vi "Resistance of the Helium Probe (Set).vi"(6 "ISOBUS address":T4=-1 caption="ISOBUS address (-1)", 8 "error in":errorcluster, 9 "Unit":T1, 10 "Resistance Configuration":T5, 11 "Mercury Reference In":T6) -> (0 "error out":errorcluster, 2 "Response":T2, 3 "Mercury Reference Out":T6, 4 "Valid?":T3)   [LabVIEW 2015, in "Mercury iXX.lvlib" / "Level Meter.lvlib"]
doc: "Set the configuration for the resistance of the helium probe at both 0% and 100%."
uses:
  Level Meter.lvlib
  Controls/Mercury Reference.ctl
  Controls/Comms Transport Layer.ctl
  Private/Controls/Query Dynamic Reference.ctl
  Controls/Resistance Configuration.ctl
  Controls/ISOBus Address.ctl
  Controls/Is Valid LED.ctl
  Controls/Response String.ctl
  Controls/Unit String.ctl
  Private/Controls/Command Verbs.ctl
  Mercury iXX.lvlib
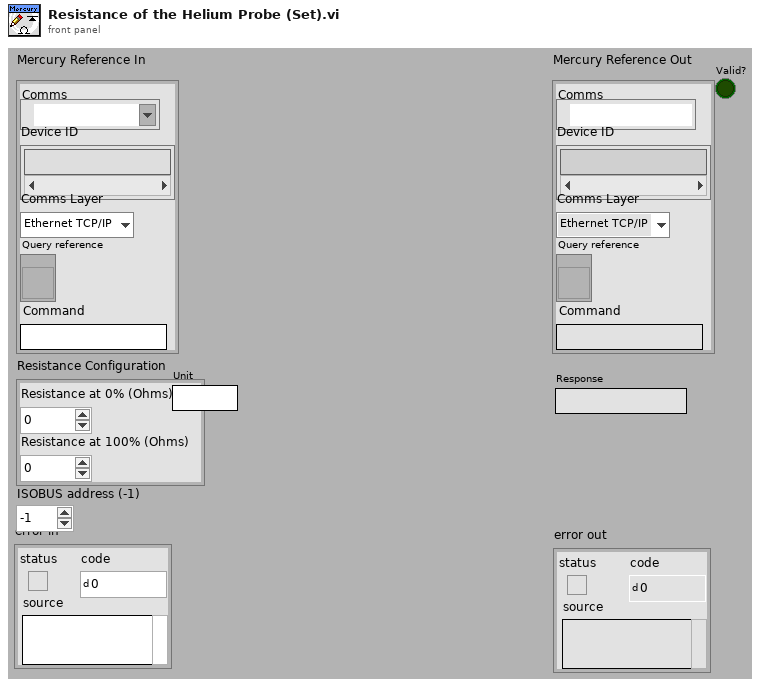
[diagram p1: front panel]
types:
  T1 = typedef "Mercury iXX.lvlib/Unit String.ctl" = string
  T2 = typedef "Mercury iXX.lvlib/Response String.ctl" = string
  T3 = typedef "Mercury iXX.lvlib/Is Valid LED.ctl" = bool
  T4 = typedef "Mercury iXX.lvlib/ISOBus Address.ctl" = i32
  T5 = typedef "Mercury iXX.lvlib/Level Meter.lvlib/Resistance Configuration.ctl" = cluster{"Res 0%":dbl, "Res 100%":dbl}
  T6 = typedef "Mercury iXX.lvlib/Mercury Reference.ctl" = cluster{"Comms":refnum<visa-resource-name>, "Device ID":string[], "Comms Layer":T7, "Command":string, "Query reference":T8}
  T7 = typedef "Mercury iXX.lvlib/Comms Transport Layer.ctl" = enum16{"Ethernet TCP/IP", "USB", "ISOBus - RS-232", "GPIB"}
  T8 = typedef "Mercury iXX.lvlib/Query Dynamic Reference.ctl" = refnum<vi>
  T9 = typedef "Mercury iXX.lvlib/Command Verbs.ctl" = string
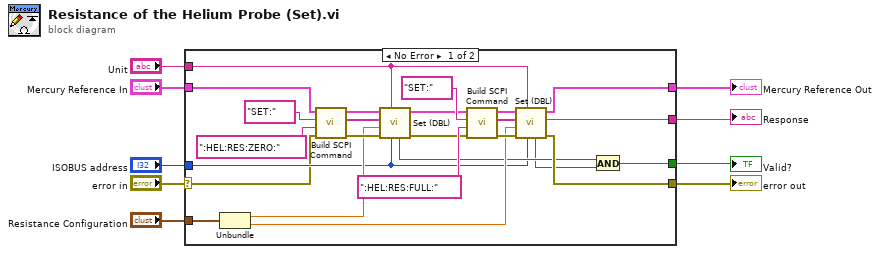
[diagram p0: block diagram]
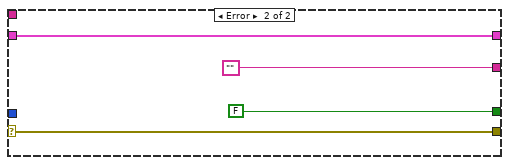
[diagram p2: hidden frame]
diagram:
  n1 = case shown="No Error" "error in" {
    selector: "error in" -> [w11 w38]
    tunnel: "Resistance Configuration" -> [w34 _]
    tunnel: "Mercury Reference In" -> [w27 w37]
    tunnel: [w18 w37] -> w7
    tunnel: [w17 w38] -> w6
    tunnel: "ISOBUS address" -> [w14 _]
    tunnel: [w13 T3 FALSE ("Valid?")] -> w4
    tunnel: [w12 ""] -> w3
    tunnel: "Unit" -> [w10 _]
    frame No Error {
      n2 = Unbundle(w34) -> ("Res 0%"=w28:dbl, "Res 100%"=w19:dbl)
      n3 = call "Build SCPI Command.vi"("error in"=w11, "Noun(s)"=":HEL:RES:ZERO:" ("Command"), "Verb"=T9 "SET:", "Mercury Reference In"=w27) -> ("error out"=w31:errorcluster, "SCPI Message(s)"=w29:string[], "Mercury Reference Out"=w30:T6)  [unwired: 5 out]
      n4 = call "Set (DBL).vi"("ISOBUS address"=w14, "Unit"=w10, "error in"=w31, "Command Value (Dbl)"=w28, "SCPI Message(s)"=w29, "Mercury Reference In"=w30) -> ("error out"=w21:errorcluster, "Mercury Reference Out"=w20:T6, "Valid?"=w16:T3)  [unwired: 3 out]
      n5 = call "Build SCPI Command.vi"("error in"=w21, "Noun(s)"=":HEL:RES:FULL:" ("Command"), "Verb"=T9 "SET:", "Mercury Reference In"=w20) -> ("error out"=w24:errorcluster, "SCPI Message(s)"=w22:string[], "Mercury Reference Out"=w23:T6)  [unwired: 5 out]
      n6 = call "Set (DBL).vi"("ISOBUS address"=w14, "Unit"=w10, "error in"=w24, "Command Value (Dbl)"=w19, "SCPI Message(s)"=w22, "Mercury Reference In"=w23) -> ("error out"=w17:errorcluster, "Response"=w12:T2, "Mercury Reference Out"=w18:T6, "Valid?"=w15:T3)  [unwired: 2 out]
      n7 = And(x=w16, y=w15) -> (x .and. y?=w13:T3)
    }
    frame Error {
    }
  }
  "Mercury Reference Out" <- w7
  "Valid?" <- w4
  "error out" <- w6
  "Response" <- w3
